vi "环动报警队列存储.vi"() -> ()   [LabVIEW 2016, in "环境动力监测库.lvlib"]
panel:
  in  "data in":T1
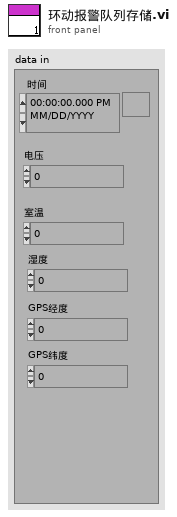
[diagram p1: front panel]
types:
  T1 = cluster{"时间":timestamp, "电压":dbl, "室温":dbl, "湿度":dbl, "GPS经度":dbl, "GPS纬度":dbl}
  T2 = cluster{"市电监测":bool, "用水量监测":bool, "烟雾监测":bool, "温度湿度":bool, "振动监测":bool, "红外入侵监测":bool, "漏水监测":bool, "门禁开关监测":bool, "门禁开关监测2":bool, "视频监测":bool, "UPS监测":bool, "空调监测":bool, "冰箱监测":bool, "排气扇监测":bool, "蓄电池监测":bool, "蓄电池监测2":bool, "GPS监测":bool, "北斗监测":bool, "气象监测":bool}
  T3 = cluster{"网络参数":cluster{"网络状态":bool, "本机IP":string[]}, "电源管理":cluster{"电源管理":bool, "氨氮电源":bool, "总磷电源":bool, "总氮电源":bool, "多参数电源":bool, "CODMn电源":bool, "CODCr电源":bool, "灯带电源":bool, "照明电源":bool}, "北斗-GPS":cluster{"GPS":cluster{"经度:":sgl, "纬度: ":sgl, "GPS监测":bool}, "北斗":cluster{"经度:":sgl, "纬度:":sgl, "北斗监测":bool}}}
  T4 = cluster{"传感器":cluster{"红外监测":cluster{"红外监测":bool, "红外入侵监测":bool}, "振动监测":cluster{"振动监测":bool, "振动监测 2":bool}, "烟雾监测":cluster{"烟雾监测":bool, "烟雾监测 2":bool}, "门禁监测":cluster{"门禁监测":bool, "门禁开关监测":bool}, "门禁2监测":cluster{"门禁监测2":bool, "门禁开关监测2":bool}, "水浸监测":cluster{"水浸监测":bool, "漏水详情":bool}}, "气象仪":cluster{"气温: ":sgl, "气压: ":sgl, "风速:":sgl, "风向:":sgl, "气象仪经度: ":sgl, "气象仪纬度: ":sgl, "详情  ":bool}}
  T5 = cluster{"市电":cluster{"状态":bool, "电压:":u16, "电流：":dbl, "详情  ":bool}, "UPS":cluster{"状态":bool, "输入电压:":sgl, "输出电压:":sgl, "电池电量:":u8, "电量":u16, "详情  ":bool}, "蓄电池12V":cluster{"状态":bool, "电压:":sgl, "电流:":sgl, "电池电量:":u8, "电量":u16, "详情  ":bool}, "蓄电池24V":cluster{"状态":bool, "电压:":sgl, "电流:":sgl, "电池电量:":u8, "电量":u16, "详情  ":bool}}
  T6 = cluster{"温湿度":cluster{"状态":bool, "温度:":sgl, "湿度:":sgl, "详情  ":bool}, "空调":cluster{"状态":bool, "机柜温度:":sgl, "压缩机:":enum16{"停止", "运行"}, "电加热:":enum16{"停止", "运行"}, "详情  ":bool}, "排气扇":cluster{"排气扇":bool, "详情  ":bool}, "冰箱":cluster{"冰箱":bool, "详情  ":bool}}
  T7 = typedef "LVDateTimeRec.ctl" = cluster{"秒数的小数部分":dbl, "秒":i32, "分":i32, "时":i32, "日":i32, "月":i32, "年":i32, "天数（周）":i32, "天数（年）":i32, "DST":i32}
  T8 = typedef "数据库类型.ctl" = enum16{"Access", "SQLite"}
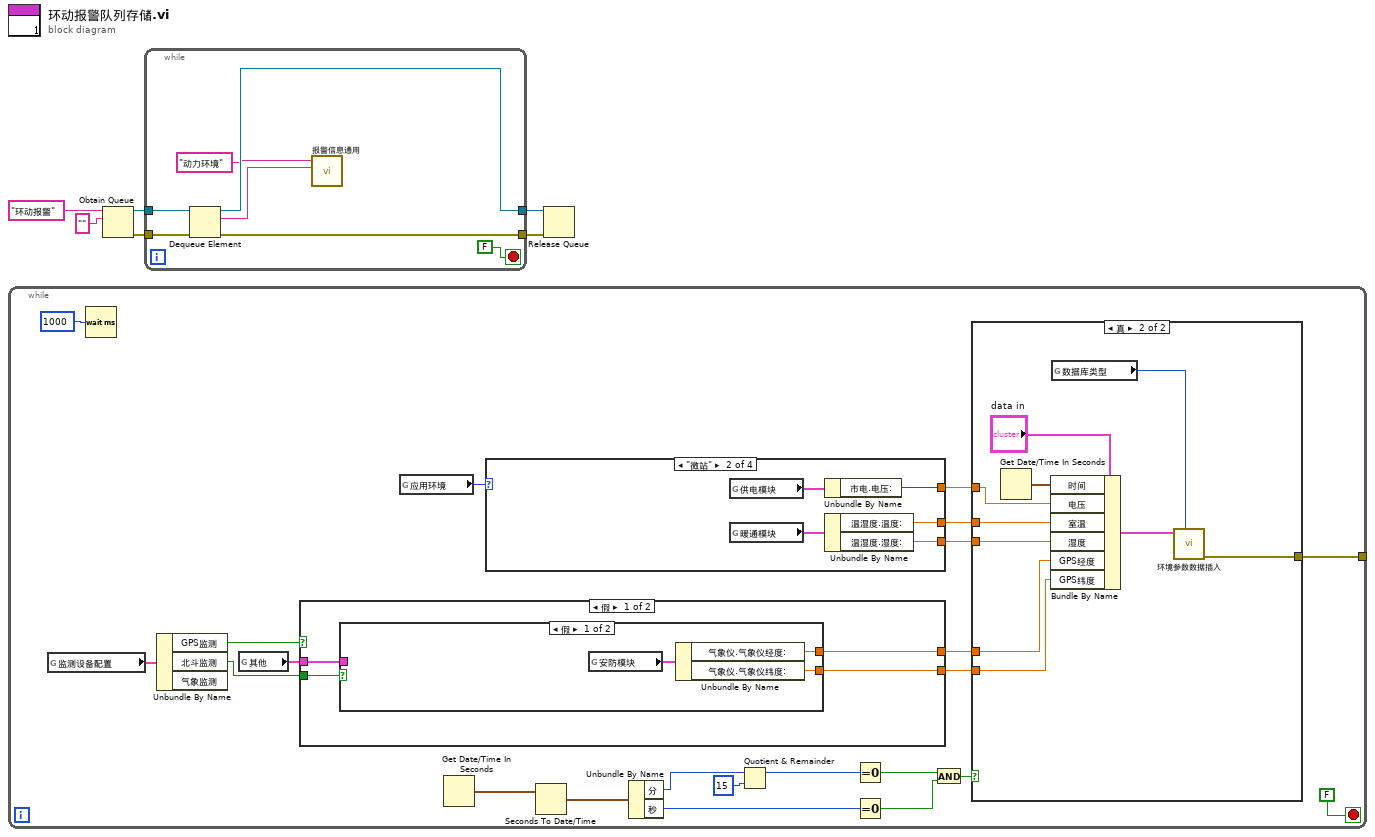
[diagram p0: block diagram]
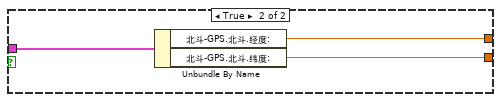
[diagram p2: hidden frame]
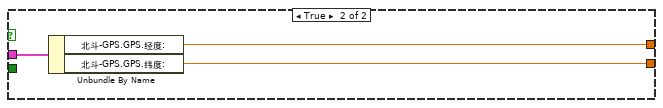
[diagram p3: hidden frame]
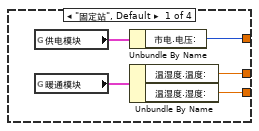
[diagram p4: hidden frame]
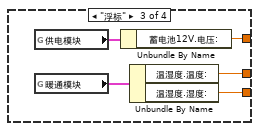
[diagram p5: hidden frame]
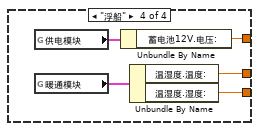
[diagram p6: hidden frame]
diagram:
  n1 = while {
    tunnel: [w26] -> _
    stop <- FALSE stop-if-true
    n2 = global read "断电保存全局变量.vi" "监测设备配置"() -> (w12:T2)
    n3 = Wait (ms)(milliseconds to wait=u32 1000 ("等待时间（毫秒）")) -> ()  [unwired: 1 out]
    n4 = Unbundle By Name(w12) -> ("GPS监测"=w11:bool, "北斗监测"=w7:bool)  [unwired: 1 out]
    n5 = global read "内部交互全局变量.vi" "其他"() -> (w10:T3)
    n6 = case shown="假" w11 {
      tunnel: w10 -> [w31 w41]
      tunnel: [w30 w40] -> w9
      tunnel: [w29 w39] -> w8
      tunnel: w7 -> [w32 _]
      frame False {
        n7 = case shown="假" w32 {
          tunnel: w31 -> [_ w36]
          tunnel: [w35 w38] -> w30
          tunnel: [w34 w37] -> w29
          frame False {
            n8 = global read "内部交互全局变量.vi" "安防模块"() -> (w33:T4)
            n9 = Unbundle By Name(w33) -> ("气象仪.气象仪经度:"=w35:sgl, "气象仪.气象仪纬度:"=w34:sgl)
          }
          frame True {
            n10 = Unbundle By Name(w36) -> ("北斗-GPS.北斗.经度:"=w38:sgl, "北斗-GPS.北斗.纬度:"=w37:sgl)
          }
        }
      }
      frame True {
        n11 = Unbundle By Name(w41) -> ("北斗-GPS.GPS.经度:"=w40:sgl, "北斗-GPS.GPS.纬度:"=w39:sgl)
      }
    }
    n12 = global read "外部交互全局变量.vi" "应用环境"() -> (w16:enum16{"固定站", "微站", "浮标", "浮船"})
    n13 = Get Date/Time In Seconds() -> (seconds since 1Jan1904=w25:timestamp)
    n14 = case shown="\"微站\"" w16 {
      tunnel: [w45 w49 w54 w59] -> w15
      tunnel: [w43 w48 w53 w58] -> w14
      tunnel: [w42 w47 w52 w57] -> w13
      frame "固定站", Default {
        n15 = global read "内部交互全局变量.vi" "供电模块"() -> (w46:T5)
        n16 = global read "内部交互全局变量.vi" "暖通模块"() -> (w44:T6)
        n17 = Unbundle By Name(w46) -> ("市电.电压:"=w45:u16)
        n18 = Unbundle By Name(w44) -> ("温湿度.温度:"=w43:sgl, "温湿度.湿度:"=w42:sgl)
      }
      frame "微站" {
        n19 = global read "内部交互全局变量.vi" "供电模块"() -> (w51:T5)
        n20 = global read "内部交互全局变量.vi" "暖通模块"() -> (w50:T6)
        n21 = Unbundle By Name(w51) -> ("市电.电压:"=w49:u16)
        n22 = Unbundle By Name(w50) -> ("温湿度.温度:"=w48:sgl, "温湿度.湿度:"=w47:sgl)
      }
      frame "浮标" {
        n23 = global read "内部交互全局变量.vi" "供电模块"() -> (w56:T5)
        n24 = global read "内部交互全局变量.vi" "暖通模块"() -> (w55:T6)
        n25 = Unbundle By Name(w56) -> ("蓄电池12V.电压:"=w54:sgl)
        n26 = Unbundle By Name(w55) -> ("温湿度.温度:"=w53:sgl, "温湿度.湿度:"=w52:sgl)
      }
      frame "浮船" {
        n27 = global read "内部交互全局变量.vi" "供电模块"() -> (w61:T5)
        n28 = global read "内部交互全局变量.vi" "暖通模块"() -> (w60:T6)
        n29 = Unbundle By Name(w61) -> ("蓄电池12V.电压:"=w59:sgl)
        n30 = Unbundle By Name(w60) -> ("温湿度.温度:"=w58:sgl, "温湿度.湿度:"=w57:sgl)
      }
    }
    n31 = Seconds To Date/Time(time stamp (now)=w25) -> (date time rec=w18:T7)  [unwired: 1 in]
    n32 = Unbundle By Name(w18) -> ("分"=w19:i32, "秒"=w22:i32)
    n33 = Quotient & Remainder(x=w19, y=15) -> (x-y*floor(x/y)=w21:i32)  [unwired: 1 out]
    n34 = Equal To 0?(x=w21) -> (x = 0?=w23:bool)
    n35 = Equal To 0?(x=w22) -> (x = 0?=w24:bool)
    n36 = And(x=w23, y=w24) -> (x .and. y?=w17:bool)
    n37 = case shown="真" w17 {
      tunnel: [_ w64] -> w26
      tunnel: w15 -> [_ w69]
      tunnel: w14 -> [_ w68]
      tunnel: w13 -> [_ w67]
      tunnel: w9 -> [_ w66]
      tunnel: w8 -> [_ w65]
      frame False {
      }
      frame True {
        n38 = Get Date/Time In Seconds() -> (seconds since 1Jan1904=w70:timestamp)
        n39 = Bundle By Name(cluster="data in", "时间"=w70, "电压"=w69, "室温"=w68, "湿度"=w67, "GPS经度"=w66, "GPS纬度"=w65) -> (w63:T1)
        n40 = global read "断电保存全局变量.vi" "数据库类型"() -> (w62:T8)
        n41 = call "环境参数数据插入.vi"("data"=w63, "数据库类型"=w62) -> ("错误输出"=w64:errorcluster)  [unwired: 8 in]
      }
    }
  }
  n42 = Obtain Queue(name (unnamed)="环动报警" ("名称（未命名）"), element data type="" ("报警内容")) -> (queue out=w6:refnum<queue>, error out=w5:errorcluster)  [unwired: 3 in, 1 out]
  n43 = while {
    tunnel: w6 -> [w78]
    tunnel: w5 -> [w77]
    tunnel: [w75] -> w3
    tunnel: [w74] -> w2
    stop <- FALSE stop-if-true
    n44 = Dequeue Element(queue=w78, error in (no error)=w77) -> (queue out=w75:refnum<queue>, element=w73:string, error out=w74:errorcluster)  [unwired: 1 in, 1 out]
    n45 = call "报警信息通用.vi"("报警信息"=w73, "设备"="动力环境") -> ()  [unwired: 9 in, 1 out]
  }
  n46 = Release Queue(queue=w3, error in (no error)=w2) -> ()  [unwired: 1 in, 3 out]
